vi "Shock&Dyanamics Laboratory - DROPBEAR_June2022_Rev3.vi"() -> ()   [LabVIEW 2019] (continued)
                n889 = property on="SG Pair Ch 18" class="Enum (strict)"("DisabledEnum"=w1070) -> ()  [unwired: 2 in, 2 out]
                n890 = property on="SG Pair Ch 16" class="Enum (strict)"("DisabledEnum"=w1072) -> ()  [unwired: 2 in, 2 out]
                n891 = property on="SG Pair Ch 19" class="Enum (strict)"("DisabledEnum"=w1069) -> ()  [unwired: 2 in, 2 out]
                n892 = property on="SG Pair Ch 26" class="Enum (strict)"("DisabledEnum"=w1061) -> ()  [unwired: 2 in, 2 out]
                n893 = property on="SG Pair Ch 17" class="Enum (strict)"("DisabledEnum"=w1071) -> ()  [unwired: 2 in, 2 out]
                n894 = property on="SG Pair Ch 24" class="Enum (strict)"("DisabledEnum"=w1059) -> ()  [unwired: 2 in, 2 out]
                n895 = property on="SG Pair Ch 27" class="Enum (strict)"("DisabledEnum"=w1062) -> ()  [unwired: 2 in, 2 out]
                n896 = property on="SG Pair Ch 25" class="Enum (strict)"("DisabledEnum"=w1060) -> ()  [unwired: 2 in, 2 out]
                n897 = property on="SG Pair Ch 22" class="Enum (strict)"("DisabledEnum"=w1057) -> ()  [unwired: 2 in, 2 out]
                n898 = property on="SG Pair Ch 30" class="Enum (strict)"("DisabledEnum"=w1065) -> ()  [unwired: 2 in, 2 out]
                n899 = property on="SG Pair Ch 31" class="Enum (strict)"("DisabledEnum"=w1066) -> ()  [unwired: 2 in, 2 out]
                n900 = property on="SG Pair Ch 23" class="Enum (strict)"("DisabledEnum"=w1058) -> ()  [unwired: 2 in, 2 out]
                n901 = property on="SG Pair Ch 28" class="Enum (strict)"("DisabledEnum"=w1063) -> ()  [unwired: 2 in, 2 out]
                n902 = property on="SG Pair Ch 29" class="Enum (strict)"("DisabledEnum"=w1064) -> ()  [unwired: 2 in, 2 out]
                n903 = property on="SG Pair Ch 20" class="Enum (strict)"("DisabledEnum"=w1055) -> ()  [unwired: 2 in, 2 out]
                n904 = property on="SG Pair Ch 21" class="Enum (strict)"("DisabledEnum"=w1056) -> ()  [unwired: 2 in, 2 out]
              }
              event "SG Pair Ch 0", "SG Pair Ch 1", "SG Pair Ch 2", "SG Pair Ch 3", "SG Pair Ch 4", "SG Pair Ch 5", "SG Pair Ch 6", "SG Pair Ch 7", "SG Pair Ch 8", "SG Pair Ch 9", "SG Pair Ch 10", "SG Pair Ch 11", "SG Pair Ch 12", "SG Pair Ch 13", "SG Pair Ch 14", "SG Pair Ch 15", "SG Pair Ch 16", "SG Pair Ch 17", "SG Pair Ch 18", "SG Pair Ch 19", "SG Pair Ch 20", "SG Pair Ch 21", "SG Pair Ch 22", "SG Pair Ch 23", "SG Pair Ch 24", "SG Pair Ch 31", "SG Pair Ch 30", "SG Pair Ch 29", "SG Pair Ch 28", "SG Pair Ch 27", "SG Pair Ch 26", "SG Pair Ch 25": Value Change {
                # "Need to prevent choosing channels to pair if they are not strain, prevent choosing same channel or channel that is already choosen\nprevent pairing channels if they are not turned on - these errors should be before execution!"
                n905 = event-data() -> ()  [unwired: 1 in, 6 out]
                n906 = property on="SG Pair Ch 29" class="Enum (strict)"() -> ("Value"=w1186:T38)  [unwired: 2 in, 2 out]
                n907 = property on="SG Pair Ch 28" class="Enum (strict)"() -> ("Value"=w1187:T37)  [unwired: 2 in, 2 out]
                n908 = property on="SG Pair Ch 31" class="Enum (strict)"() -> ("Value"=w1184:T40)  [unwired: 2 in, 2 out]
                n909 = property on="SG Pair Ch 25" class="Enum (strict)"() -> ("Value"=w1190:T34)  [unwired: 2 in, 2 out]
                n910 = property on="SG Pair Ch 30" class="Enum (strict)"() -> ("Value"=w1185:T39)  [unwired: 2 in, 2 out]
                n911 = property on="SG Pair Ch 24" class="Enum (strict)"() -> ("Value"=w1191:T33)  [unwired: 2 in, 2 out]
                n912 = property on="SG Pair Ch 27" class="Enum (strict)"() -> ("Value"=w1188:T36)  [unwired: 2 in, 2 out]
                n913 = property on="SG Pair Ch 21" class="Enum (strict)"() -> ("Value"=w1194:T30)  [unwired: 2 in, 2 out]
                n914 = property on="SG Pair Ch 26" class="Enum (strict)"() -> ("Value"=w1189:T35)  [unwired: 2 in, 2 out]
                n915 = property on="SG Pair Ch 20" class="Enum (strict)"() -> ("Value"=w1195:T29)  [unwired: 2 in, 2 out]
                n916 = property on="SG Pair Ch 23" class="Enum (strict)"() -> ("Value"=w1192:T32)  [unwired: 2 in, 2 out]
                n917 = property on="SG Pair Ch 13" class="Enum (strict)"() -> ("Value"=w1202:T22)  [unwired: 2 in, 2 out]
                n918 = property on="SG Pair Ch 17" class="Enum (strict)"() -> ("Value"=w1198:T26)  [unwired: 2 in, 2 out]
                n919 = property on="SG Pair Ch 22" class="Enum (strict)"() -> ("Value"=w1193:T31)  [unwired: 2 in, 2 out]
                n920 = property on="SG Pair Ch 12" class="Enum (strict)"() -> ("Value"=w1203:T21)  [unwired: 2 in, 2 out]
                n921 = property on="SG Pair Ch 15" class="Enum (strict)"() -> ("Value"=w1200:T24)  [unwired: 2 in, 2 out]
                n922 = property on="SG Pair Ch 16" class="Enum (strict)"() -> ("Value"=w1199:T25)  [unwired: 2 in, 2 out]
                n923 = property on="SG Pair Ch 19" class="Enum (strict)"() -> ("Value"=w1196:T28)  [unwired: 2 in, 2 out]
                n924 = property on="SG Pair Ch 9" class="Enum (strict)"() -> ("Value"=w1206:T18)  [unwired: 2 in, 2 out]
                n925 = property on="SG Pair Ch 14" class="Enum (strict)"() -> ("Value"=w1201:T23)  [unwired: 2 in, 2 out]
                n926 = property on="SG Pair Ch 18" class="Enum (strict)"() -> ("Value"=w1197:T27)  [unwired: 2 in, 2 out]
                n927 = property on="SG Pair Ch 8" class="Enum (strict)"() -> ("Value"=w1207:T17)  [unwired: 2 in, 2 out]
                n928 = property on="SG Pair Ch 11" class="Enum (strict)"() -> ("Value"=w1204:T20)  [unwired: 2 in, 2 out]
                n929 = property on="SG Pair Ch 5" class="Enum (strict)"() -> ("Value"=w1210:T14)  [unwired: 2 in, 2 out]
                n930 = property on="SG Pair Ch 10" class="Enum (strict)"() -> ("Value"=w1205:T19)  [unwired: 2 in, 2 out]
                n931 = property on="SG Pair Ch 4" class="Enum (strict)"() -> ("Value"=w1211:T13)  [unwired: 2 in, 2 out]
                n932 = property on="SG Pair Ch 7" class="Enum (strict)"() -> ("Value"=w1208:T16)  [unwired: 2 in, 2 out]
                n933 = property on="SG Pair Ch 1" class="Enum (strict)"() -> ("Value"=w1214:T10)  [unwired: 2 in, 2 out]
                n934 = property on="SG Pair Ch 6" class="Enum (strict)"() -> ("Value"=w1209:T15)  [unwired: 2 in, 2 out]
                n935 = property on="SG Pair Ch 0" class="Enum (strict)"() -> ("Value"=w1215:T9)  [unwired: 2 in, 2 out]
                n936 = property on="SG Pair Ch 3" class="Enum (strict)"() -> ("Value"=w1212:T12)  [unwired: 2 in, 2 out]
                n937 = property on="SG Pair Ch 2" class="Enum (strict)"() -> ("Value"=w1213:T11)  [unwired: 2 in, 2 out]
                n938 = Build Array(w1215, w1214, w1213, w1212, w1211, w1210, w1209, w1208, w1207, w1206, w1205, w1204, w1203, w1202, w1201, w1200, w1199, w1198, w1197, w1196, w1195, w1194, w1193, w1192, w1191, w1190, w1189, w1188, w1187, w1186, w1185, w1184) -> (w1217:u16[])
                n939 = for {
                  tunnel: w1217 -> [w1218] mode=indexing
                  i -> [w1219]
                  n940 = Equal?(x=w1219, y=w1218) -> (x = y?=w1221:bool)
                  n941 = Not(x=w1221) -> (.not. x?=w1220:bool)
                  n942 = case shown="True" w1220 {
                    tunnel: w1219 -> [_ w1224]
                    tunnel: w1218 -> [_ w1223]
                    frame False {
                      # "Add error here - cannot pair a Strain Channel with itself"
                      n943 = One Button Dialog(message="The Strain channel cannot be paired with itself. \nPlease select a different channel.") -> ()  [unwired: 1 in, 1 out]
                    }
                    frame True {
                      n944 = case shown="33" w1223 {
                        tunnel: T42."Disabled and Grayed Out" ("Disabled") -> [w1228 w1230 w1233 w1236 w1239 w1242 w1245 w1248 w1251 w1254 w1257 w1260 w1263 w1266 w1269 w1272 w1275 w1278 w1281 w1284 w1287 w1290 w1293 w1296 w1299 w1302 w1305 w1308 w1311 w1314 w1317 w1320 _ _]
                        tunnel: w1224 -> [w1227 w1229 w1232 w1235 w1238 w1241 w1244 w1247 w1250 w1253 w1256 w1259 w1262 w1265 w1268 w1271 w1274 w1277 w1280 w1283 w1286 w1289 w1292 w1295 w1298 w1301 w1304 w1307 w1310 w1313 w1316 w1319 _ _]
                        frame 0, Default {
                          n945 = property on="SG Pair Ch 0" class="Enum (strict)"("Value"=w1227) -> (error out=w1226:errorcluster)  [unwired: 2 in, 1 out]
                          n946 = property on="SG Pair Ch 0" class="Enum (strict)"(error in=w1226, "DisabledEnum"=w1228) -> ()  [unwired: 1 in, 2 out]
                        }
                        frame 1 {
                          n947 = property on="SG Pair Ch 1" class="Enum (strict)"("Value"=w1229) -> (error out=w1231:errorcluster)  [unwired: 2 in, 1 out]
                          n948 = property on="SG Pair Ch 1" class="Enum (strict)"(error in=w1231, "DisabledEnum"=w1230) -> ()  [unwired: 1 in, 2 out]
                        }
                        frame 2 {
                          n949 = property on="SG Pair Ch 2" class="Enum (strict)"("Value"=w1232) -> (error out=w1234:errorcluster)  [unwired: 2 in, 1 out]
                          n950 = property on="SG Pair Ch 2" class="Enum (strict)"(error in=w1234, "DisabledEnum"=w1233) -> ()  [unwired: 1 in, 2 out]
                        }
                        frame 3 {
                          n951 = property on="SG Pair Ch 3" class="Enum (strict)"("Value"=w1235) -> (error out=w1237:errorcluster)  [unwired: 2 in, 1 out]
                          n952 = property on="SG Pair Ch 3" class="Enum (strict)"(error in=w1237, "DisabledEnum"=w1236) -> ()  [unwired: 1 in, 2 out]
                        }
                        frame 4 {
                          n953 = property on="SG Pair Ch 4" class="Enum (strict)"("Value"=w1238) -> (error out=w1240:errorcluster)  [unwired: 2 in, 1 out]
                          n954 = property on="SG Pair Ch 4" class="Enum (strict)"(error in=w1240, "DisabledEnum"=w1239) -> ()  [unwired: 1 in, 2 out]
                        }
                        frame 5 {
                          n955 = property on="SG Pair Ch 5" class="Enum (strict)"("Value"=w1241) -> (error out=w1243:errorcluster)  [unwired: 2 in, 1 out]
                          n956 = property on="SG Pair Ch 5" class="Enum (strict)"(error in=w1243, "DisabledEnum"=w1242) -> ()  [unwired: 1 in, 2 out]
                        }
                        frame 6 {
                          n957 = property on="SG Pair Ch 6" class="Enum (strict)"("Value"=w1244) -> (error out=w1246:errorcluster)  [unwired: 2 in, 1 out]
                          n958 = property on="SG Pair Ch 6" class="Enum (strict)"(error in=w1246, "DisabledEnum"=w1245) -> ()  [unwired: 1 in, 2 out]
                        }
                        frame 7 {
                          n959 = property on="SG Pair Ch 7" class="Enum (strict)"("Value"=w1247) -> (error out=w1249:errorcluster)  [unwired: 2 in, 1 out]
                          n960 = property on="SG Pair Ch 7" class="Enum (strict)"(error in=w1249, "DisabledEnum"=w1248) -> ()  [unwired: 1 in, 2 out]
                        }
                        frame 8 {
                          n961 = property on="SG Pair Ch 8" class="Enum (strict)"("Value"=w1250) -> (error out=w1252:errorcluster)  [unwired: 2 in, 1 out]
                          n962 = property on="SG Pair Ch 8" class="Enum (strict)"(error in=w1252, "DisabledEnum"=w1251) -> ()  [unwired: 1 in, 2 out]
                        }
                        frame 9 {
                          n963 = property on="SG Pair Ch 9" class="Enum (strict)"("Value"=w1253) -> (error out=w1255:errorcluster)  [unwired: 2 in, 1 out]
                          n964 = property on="SG Pair Ch 9" class="Enum (strict)"(error in=w1255, "DisabledEnum"=w1254) -> ()  [unwired: 1 in, 2 out]
                        }
                        frame 10 {
                          n965 = property on="SG Pair Ch 10" class="Enum (strict)"("Value"=w1256) -> (error out=w1258:errorcluster)  [unwired: 2 in, 1 out]
                          n966 = property on="SG Pair Ch 10" class="Enum (strict)"(error in=w1258, "DisabledEnum"=w1257) -> ()  [unwired: 1 in, 2 out]
                        }
                        frame 11 {
                          n967 = property on="SG Pair Ch 11" class="Enum (strict)"("Value"=w1259) -> (error out=w1261:errorcluster)  [unwired: 2 in, 1 out]
                          n968 = property on="SG Pair Ch 11" class="Enum (strict)"(error in=w1261, "DisabledEnum"=w1260) -> ()  [unwired: 1 in, 2 out]
                        }
                        frame 12 {
                          n969 = property on="SG Pair Ch 12" class="Enum (strict)"("Value"=w1262) -> (error out=w1264:errorcluster)  [unwired: 2 in, 1 out]
                          n970 = property on="SG Pair Ch 12" class="Enum (strict)"(error in=w1264, "DisabledEnum"=w1263) -> ()  [unwired: 1 in, 2 out]
                        }
                        frame 13 {
                          n971 = property on="SG Pair Ch 13" class="Enum (strict)"("Value"=w1265) -> (error out=w1267:errorcluster)  [unwired: 2 in, 1 out]
                          n972 = property on="SG Pair Ch 13" class="Enum (strict)"(error in=w1267, "DisabledEnum"=w1266) -> ()  [unwired: 1 in, 2 out]
                        }
                        frame 14 {
                          n973 = property on="SG Pair Ch 14" class="Enum (strict)"("Value"=w1268) -> (error out=w1270:errorcluster)  [unwired: 2 in, 1 out]
                          n974 = property on="SG Pair Ch 14" class="Enum (strict)"(error in=w1270, "DisabledEnum"=w1269) -> ()  [unwired: 1 in, 2 out]
                        }
                        frame 15 {
                          n975 = property on="SG Pair Ch 15" class="Enum (strict)"("Value"=w1271) -> (error out=w1273:errorcluster)  [unwired: 2 in, 1 out]
                          n976 = property on="SG Pair Ch 15" class="Enum (strict)"(error in=w1273, "DisabledEnum"=w1272) -> ()  [unwired: 1 in, 2 out]
                        }
                        frame 16 {
                          n977 = property on="SG Pair Ch 16" class="Enum (strict)"("Value"=w1274) -> (error out=w1276:errorcluster)  [unwired: 2 in, 1 out]
                          n978 = property on="SG Pair Ch 16" class="Enum (strict)"(error in=w1276, "DisabledEnum"=w1275) -> ()  [unwired: 1 in, 2 out]
                        }
                        frame 17 {
                          n979 = property on="SG Pair Ch 17" class="Enum (strict)"("Value"=w1277) -> (error out=w1279:errorcluster)  [unwired: 2 in, 1 out]
                          n980 = property on="SG Pair Ch 17" class="Enum (strict)"(error in=w1279, "DisabledEnum"=w1278) -> ()  [unwired: 1 in, 2 out]
                        }
                        frame 18 {
                          n981 = property on="SG Pair Ch 18" class="Enum (strict)"("Value"=w1280) -> (error out=w1282:errorcluster)  [unwired: 2 in, 1 out]
                          n982 = property on="SG Pair Ch 18" class="Enum (strict)"(error in=w1282, "DisabledEnum"=w1281) -> ()  [unwired: 1 in, 2 out]
                        }
                        frame 19 {
                          n983 = property on="SG Pair Ch 19" class="Enum (strict)"("Value"=w1283) -> (error out=w1285:errorcluster)  [unwired: 2 in, 1 out]
                          n984 = property on="SG Pair Ch 19" class="Enum (strict)"(error in=w1285, "DisabledEnum"=w1284) -> ()  [unwired: 1 in, 2 out]
                        }
                        frame 20 {
                          n985 = property on="SG Pair Ch 20" class="Enum (strict)"("Value"=w1286) -> (error out=w1288:errorcluster)  [unwired: 2 in, 1 out]
                          n986 = property on="SG Pair Ch 20" class="Enum (strict)"(error in=w1288, "DisabledEnum"=w1287) -> ()  [unwired: 1 in, 2 out]
                        }
                        frame 21 {
                          n987 = property on="SG Pair Ch 21" class="Enum (strict)"("Value"=w1289) -> (error out=w1291:errorcluster)  [unwired: 2 in, 1 out]
                          n988 = property on="SG Pair Ch 21" class="Enum (strict)"(error in=w1291, "DisabledEnum"=w1290) -> ()  [unwired: 1 in, 2 out]
                        }
                        frame 22 {
                          n989 = property on="SG Pair Ch 22" class="Enum (strict)"("Value"=w1292) -> (error out=w1294:errorcluster)  [unwired: 2 in, 1 out]
                          n990 = property on="SG Pair Ch 22" class="Enum (strict)"(error in=w1294, "DisabledEnum"=w1293) -> ()  [unwired: 1 in, 2 out]
                        }
                        frame 23 {
                          n991 = property on="SG Pair Ch 23" class="Enum (strict)"("Value"=w1295) -> (error out=w1297:errorcluster)  [unwired: 2 in, 1 out]
                          n992 = property on="SG Pair Ch 23" class="Enum (strict)"(error in=w1297, "DisabledEnum"=w1296) -> ()  [unwired: 1 in, 2 out]
                        }
                        frame 24 {
                          n993 = property on="SG Pair Ch 24" class="Enum (strict)"("Value"=w1298) -> (error out=w1300:errorcluster)  [unwired: 2 in, 1 out]
                          n994 = property on="SG Pair Ch 24" class="Enum (strict)"(error in=w1300, "DisabledEnum"=w1299) -> ()  [unwired: 1 in, 2 out]
                        }
                        frame 25 {
                          n995 = property on="SG Pair Ch 25" class="Enum (strict)"("Value"=w1301) -> (error out=w1303:errorcluster)  [unwired: 2 in, 1 out]
                          n996 = property on="SG Pair Ch 25" class="Enum (strict)"(error in=w1303, "DisabledEnum"=w1302) -> ()  [unwired: 1 in, 2 out]
                        }
                        frame 26 {
                          n997 = property on="SG Pair Ch 26" class="Enum (strict)"("Value"=w1304) -> (error out=w1306:errorcluster)  [unwired: 2 in, 1 out]
                          n998 = property on="SG Pair Ch 26" class="Enum (strict)"(error in=w1306, "DisabledEnum"=w1305) -> ()  [unwired: 1 in, 2 out]
                        }
                        frame 27 {
                          n999 = property on="SG Pair Ch 27" class="Enum (strict)"("Value"=w1307) -> (error out=w1309:errorcluster)  [unwired: 2 in, 1 out]
                          n1000 = property on="SG Pair Ch 27" class="Enum (strict)"(error in=w1309, "DisabledEnum"=w1308) -> ()  [unwired: 1 in, 2 out]
                        }
                        frame 28 {
                          n1001 = property on="SG Pair Ch 28" class="Enum (strict)"("Value"=w1310) -> (error out=w1312:errorcluster)  [unwired: 2 in, 1 out]
                          n1002 = property on="SG Pair Ch 28" class="Enum (strict)"(error in=w1312, "DisabledEnum"=w1311) -> ()  [unwired: 1 in, 2 out]
                        }
                        frame 29 {
                          n1003 = property on="SG Pair Ch 29" class="Enum (strict)"("Value"=w1313) -> (error out=w1315:errorcluster)  [unwired: 2 in, 1 out]
                          n1004 = property on="SG Pair Ch 29" class="Enum (strict)"(error in=w1315, "DisabledEnum"=w1314) -> ()  [unwired: 1 in, 2 out]
                        }
                        frame 30 {
                          n1005 = property on="SG Pair Ch 30" class="Enum (strict)"("Value"=w1316) -> (error out=w1318:errorcluster)  [unwired: 2 in, 1 out]
                          n1006 = property on="SG Pair Ch 30" class="Enum (strict)"(error in=w1318, "DisabledEnum"=w1317) -> ()  [unwired: 1 in, 2 out]
                        }
                        frame 31 {
                          n1007 = property on="SG Pair Ch 31" class="Enum (strict)"("Value"=w1319) -> (error out=w1321:errorcluster)  [unwired: 2 in, 1 out]
                          n1008 = property on="SG Pair Ch 31" class="Enum (strict)"(error in=w1321, "DisabledEnum"=w1320) -> ()  [unwired: 1 in, 2 out]
                        }
                        frame 32 {
                        }
                        frame 33 {
                        }
                      }
                    }
                  }
                }
              }
              event "Signal Type 0", "Signal Type 1", "Signal Type 2", "Signal Type 3", "Signal Type 4", "Signal Type 5", "Signal Type 6", "Signal Type 7", "Signal Type 8", "Signal Type 9", "Signal Type 10", "Signal Type 11", "Signal Type 12", "Signal Type 13", "Signal Type 14", "Signal Type 15", "Signal Type 16", "Signal Type 17", "Signal Type 18", "Signal Type 19", "Signal Type 20", "Signal Type 21", "Signal Type 22", "Signal Type 23", "Signal Type 24", "Signal Type 25", "Signal Type 26", "Signal Type 27", "Signal Type 28", "Signal Type 29", "Signal Type 30", "Signal Type 31": Value Change {
                n1009 = event-data() -> ()  [unwired: 1 in, 5 out]
                n1010 = property on="Signal Type 23" class="Enum (strict)"() -> ("Value"=w1346:T8)  [unwired: 2 in, 2 out]
                n1011 = property on="Signal Type 21" class="Enum (strict)"() -> ("Value"=w1348:T8)  [unwired: 2 in, 2 out]
                n1012 = property on="Signal Type 20" class="Enum (strict)"() -> ("Value"=w1349:T8)  [unwired: 2 in, 2 out]
                n1013 = property on="Signal Type 22" class="Enum (strict)"() -> ("Value"=w1347:T8)  [unwired: 2 in, 2 out]
                n1014 = property on="Signal Type 26" class="Enum (strict)"() -> ("Value"=w1343:T8)  [unwired: 2 in, 2 out]
                n1015 = property on="Signal Type 1" class="Enum (strict)"() -> ("Value"=w1384:T8)  [unwired: 2 in, 2 out]
                n1016 = property on="Signal Type 6" class="Enum (strict)"() -> ("Value"=w1376:T8)  [unwired: 2 in, 2 out]
                n1017 = property on="Signal Type 7" class="Enum (strict)"() -> ("Value"=w1375:T8)  [unwired: 2 in, 2 out]
                n1018 = property on="Signal Type 19" class="Enum (strict)"() -> ("Value"=w1350:T8)  [unwired: 2 in, 2 out]
                n1019 = property on="Signal Type 5" class="Enum (strict)"() -> ("Value"=w1377:T8)  [unwired: 2 in, 2 out]
                n1020 = property on="Signal Type 0" class="Enum (strict)"() -> ("Value"=w1386:T8)  [unwired: 2 in, 2 out]
                n1021 = property on="Signal Type 2" class="Enum (strict)"() -> ("Value"=w1383:T8)  [unwired: 2 in, 2 out]
                n1022 = property on="Signal Type 3" class="Enum (strict)"() -> ("Value"=w1380:T8)  [unwired: 2 in, 2 out]
                n1023 = property on="Signal Type 4" class="Enum (strict)"() -> ("Value"=w1378:T8)  [unwired: 2 in, 2 out]
                n1024 = property on="Signal Type 9" class="Enum (strict)"() -> ("Value"=w1366:T8)  [unwired: 2 in, 2 out]
                n1025 = property on="Signal Type 8" class="Enum (strict)"() -> ("Value"=w1367:T8)  [unwired: 2 in, 2 out]
                n1026 = property on="Signal Type 13" class="Enum (strict)"() -> ("Value"=w1357:T8)  [unwired: 2 in, 2 out]
                n1027 = property on="Signal Type 30" class="Enum (strict)"() -> ("Value"=w1338:T8)  [unwired: 2 in, 2 out]
                n1028 = property on="Signal Type 10" class="Enum (strict)"() -> ("Value"=w1365:T8)  [unwired: 2 in, 2 out]
                n1029 = property on="Signal Type 25" class="Enum (strict)"() -> ("Value"=w1344:T8)  [unwired: 2 in, 2 out]
                n1030 = property on="Signal Type 29" class="Enum (strict)"() -> ("Value"=w1340:T8)  [unwired: 2 in, 2 out]
                n1031 = property on="Signal Type 11" class="Enum (strict)"() -> ("Value"=w1359:T8)  [unwired: 2 in, 2 out]
                n1032 = property on="Signal Type 12" class="Enum (strict)"() -> ("Value"=w1358:T8)  [unwired: 2 in, 2 out]
                n1033 = property on="Signal Type 24" class="Enum (strict)"() -> ("Value"=w1345:T8)  [unwired: 2 in, 2 out]
                n1034 = property on="Signal Type 15" class="Enum (strict)"() -> ("Value"=w1355:T8)  [unwired: 2 in, 2 out]
                n1035 = property on="Signal Type 31" class="Enum (strict)"() -> ("Value"=w1339:T8)  [unwired: 2 in, 2 out]
                n1036 = property on="Signal Type 27" class="Enum (strict)"() -> ("Value"=w1342:T8)  [unwired: 2 in, 2 out]
                n1037 = property on="Signal Type 16" class="Enum (strict)"() -> ("Value"=w1353:T8)  [unwired: 2 in, 2 out]
                n1038 = property on="Signal Type 17" class="Enum (strict)"() -> ("Value"=w1352:T8)  [unwired: 2 in, 2 out]
                n1039 = property on="Signal Type 18" class="Enum (strict)"() -> ("Value"=w1351:T8)  [unwired: 2 in, 2 out]
                n1040 = property on="Signal Type 14" class="Enum (strict)"() -> ("Value"=w1356:T8)  [unwired: 2 in, 2 out]
                n1041 = property on="Signal Type 28" class="Enum (strict)"() -> ("Value"=w1341:T8)  [unwired: 2 in, 2 out]
                n1042 = case shown="\"Voltage\", Default" w1338 {
                  tunnel: [T42."Enabled" ("Disabled") T42."Disabled and Grayed Out" ("Disabled")] -> w1324
                  frame "Strain" {
                    n1043 = property on="SG Pair 30" class="Bool (strict)"() -> ("Value"=w1392:bool)  [unwired: 2 in, 2 out]
                    n1044 = case shown="True" w1392 {
                      tunnel: [T42."Disabled and Grayed Out" ("Disabled") T42."Enabled" ("Disabled")] -> _
                      frame False {
                      }
                      frame True {
                      }
                    }
                  }
                  frame "Voltage", Default {
                  }
                }
                n1045 = case shown="\"Voltage\", Default" w1339 {
                  tunnel: [T42."Enabled" ("Disabled") T42."Disabled and Grayed Out" ("Disabled")] -> w1325
                  frame "Strain" {
                    n1046 = property on="SG Pair 31" class="Bool (strict)"() -> ("Value"=w1387:bool)  [unwired: 2 in, 2 out]
                    n1047 = case shown="True" w1387 {
                      tunnel: [T42."Disabled and Grayed Out" ("Disabled") T42."Enabled" ("Disabled")] -> _
                      frame False {
                      }
                      frame True {
                      }
                    }
                  }
                  frame "Voltage", Default {
                  }
                }
                n1048 = case shown="\"Voltage\", Default" w1340 {
                  tunnel: [T42."Enabled" ("Disabled") T42."Disabled and Grayed Out" ("Disabled")] -> w1323
                  frame "Strain" {
                    n1049 = property on="SG Pair 29" class="Bool (strict)"() -> ("Value"=w1397:bool)  [unwired: 2 in, 2 out]
                    n1050 = case shown="True" w1397 {
                      tunnel: [T42."Disabled and Grayed Out" ("Disabled") T42."Enabled" ("Disabled")] -> _
                      frame False {
                      }
                      frame True {
                      }
                    }
                  }
                  frame "Voltage", Default {
                  }
                }
                n1051 = case shown="\"Strain\"" w1342 {
                  tunnel: [T42."Enabled" ("Disabled") T42."Disabled and Grayed Out" ("Disabled")] -> w1326
                  frame "Strain" {
                    n1052 = property on="SG Pair 27" class="Bool (strict)"() -> ("Value"=w1407:bool)  [unwired: 2 in, 2 out]
                    n1053 = case shown="True" w1407 {
                      tunnel: [T42."Disabled and Grayed Out" ("Disabled") T42."Enabled" ("Disabled")] -> _
                      frame False {
                      }
                      frame True {
                      }
                    }
                  }
                  frame "Voltage", Default {
                  }
                }
                n1054 = case shown="\"Voltage\", Default" w1341 {
                  tunnel: [T42."Enabled" ("Disabled") T42."Disabled and Grayed Out" ("Disabled")] -> w1322
                  frame "Strain" {
                    n1055 = property on="SG Pair 28" class="Bool (strict)"() -> ("Value"=w1402:bool)  [unwired: 2 in, 2 out]
                    n1056 = case shown="True" w1402 {
                      tunnel: [T42."Disabled and Grayed Out" ("Disabled") T42."Enabled" ("Disabled")] -> _
                      frame False {
                      }
                      frame True {
                      }
                    }
                  }
                  frame "Voltage", Default {
                  }
                }
                n1057 = case shown="\"Strain\"" w1343 {
                  tunnel: [T42."Enabled" ("Disabled") T42."Disabled and Grayed Out" ("Disabled")] -> w1327
                  frame "Strain" {
                    n1058 = property on="SG Pair 26" class="Bool (strict)"() -> ("Value"=w1412:bool)  [unwired: 2 in, 2 out]
                    n1059 = case shown="True" w1412 {
                      tunnel: [T42."Disabled and Grayed Out" ("Disabled") T42."Enabled" ("Disabled")] -> _
                      frame False {
                      }
                      frame True {
                      }
                    }
                  }
                  frame "Voltage", Default {
                  }
                }
                n1060 = case shown="\"Voltage\", Default" w1344 {
                  tunnel: [T42."Enabled" ("Disabled") T42."Disabled and Grayed Out" ("Disabled")] -> w1328
                  frame "Strain" {
                    n1061 = property on="SG Pair 25" class="Bool (strict)"() -> ("Value"=w1417:bool)  [unwired: 2 in, 2 out]
                    n1062 = case shown="True" w1417 {
                      tunnel: [T42."Disabled and Grayed Out" ("Disabled") T42."Enabled" ("Disabled")] -> _
                      frame False {
                      }
                      frame True {
                      }
                    }
                  }
                  frame "Voltage", Default {
                  }
                }
                n1063 = case shown="\"Strain\"" w1366 {
                  tunnel: [T42."Enabled" ("Disabled") T42."Disabled and Grayed Out" ("Disabled")] -> w1369
                  frame "Strain" {
                    n1064 = property on="SG Pair 9" class="Bool (strict)"() -> ("Value"=w1497:bool)  [unwired: 2 in, 2 out]
                    n1065 = case shown="True" w1497 {
                      tunnel: [T42."Disabled and Grayed Out" ("Disabled") T42."Enabled" ("Disabled")] -> _
                      frame False {
                      }
                      frame True {
                      }
                    }
                  }
                  frame "Voltage", Default {
                  }
                }
                n1066 = case shown="\"Voltage\", Default" w1345 {
                  tunnel: [T42."Enabled" ("Disabled") T42."Disabled and Grayed Out" ("Disabled")] -> w1329
                  frame "Strain" {
                    n1067 = property on="SG Pair 24" class="Bool (strict)"() -> ("Value"=w1422:bool)  [unwired: 2 in, 2 out]
                    n1068 = case shown="True" w1422 {
                      tunnel: [T42."Disabled and Grayed Out" ("Disabled") T42."Enabled" ("Disabled")] -> _
                      frame False {
                      }
                      frame True {
                      }
                    }
                  }
                  frame "Voltage", Default {
                  }
                }
                n1069 = case shown="\"Strain\"" w1367 {
                  tunnel: [T42."Enabled" ("Disabled") T42."Disabled and Grayed Out" ("Disabled")] -> w1370
                  frame "Strain" {
                    n1070 = property on="SG Pair 8" class="Bool (strict)"() -> ("Value"=w1502:bool)  [unwired: 2 in, 2 out]
                    n1071 = case shown="True" w1502 {
                      tunnel: [T42."Disabled and Grayed Out" ("Disabled") T42."Enabled" ("Disabled")] -> _
                      frame False {
                      }
                      frame True {
                      }
                    }
                  }
                  frame "Voltage", Default {
                  }
                }
                n1072 = case shown="\"Voltage\", Default" w1346 {
                  tunnel: [T42."Enabled" ("Disabled") T42."Disabled and Grayed Out" ("Disabled")] -> w1330
                  frame "Strain" {
                    n1073 = property on="SG Pair 23" class="Bool (strict)"() -> ("Value"=w1427:bool)  [unwired: 2 in, 2 out]
                    n1074 = case shown="True" w1427 {
                      tunnel: [T42."Disabled and Grayed Out" ("Disabled") T42."Enabled" ("Disabled")] -> _
                      frame False {
                      }
                      frame True {
                      }
                    }
                  }
                  frame "Voltage", Default {
                  }
                }
                n1075 = case shown="\"Strain\"" w1378 {
                  tunnel: [T42."Enabled" ("Disabled") T42."Disabled and Grayed Out" ("Disabled")] -> w1371
                  frame "Strain" {
                    n1076 = property on="SG Pair 4" class="Bool (strict)"() -> ("Value"=w1522:bool)  [unwired: 2 in, 2 out]
                    n1077 = case shown="True" w1522 {
                      tunnel: [T42."Disabled and Grayed Out" ("Disabled") T42."Enabled" ("Disabled")] -> _
                      frame False {
                      }
                      frame True {
                      }
                    }
                  }
                  frame "Voltage", Default {
                  }
                }
                n1078 = case shown="\"Strain\"" w1377 {
                  tunnel: [T42."Enabled" ("Disabled") T42."Disabled and Grayed Out" ("Disabled")] -> w1372
                  frame "Strain" {
                    n1079 = property on="SG Pair 5" class="Bool (strict)"() -> ("Value"=w1517:bool)  [unwired: 2 in, 2 out]
                    n1080 = case shown="True" w1517 {
                      tunnel: [T42."Disabled and Grayed Out" ("Disabled") T42."Enabled" ("Disabled")] -> _
                      frame False {
                      }
                      frame True {
                      }
                    }
                  }
                  frame "Voltage", Default {
                  }
                }
                n1081 = case shown="\"Strain\"" w1375 {
                  tunnel: [T42."Enabled" ("Disabled") T42."Disabled and Grayed Out" ("Disabled")] -> w1374
                  frame "Strain" {
                    n1082 = property on="SG Pair 7" class="Bool (strict)"() -> ("Value"=w1507:bool)  [unwired: 2 in, 2 out]
                    n1083 = case shown="True" w1507 {
                      tunnel: [T42."Disabled and Grayed Out" ("Disabled") T42."Enabled" ("Disabled")] -> _
                      frame False {
                      }
                      frame True {
                      }
                    }
                  }
                  frame "Voltage", Default {
                  }
                }
                n1084 = case shown="\"Strain\"" w1358 {
                  tunnel: [T42."Enabled" ("Disabled") T42."Disabled and Grayed Out" ("Disabled")] -> w1363
                  frame "Strain" {
                    n1085 = property on="SG Pair 12" class="Bool (strict)"() -> ("Value"=w1482:bool)  [unwired: 2 in, 2 out]
                    n1086 = case shown="True" w1482 {
                      tunnel: [T42."Disabled and Grayed Out" ("Disabled") T42."Enabled" ("Disabled")] -> _
                      frame False {
                      }
                      frame True {
                      }
                    }
                  }
                  frame "Voltage", Default {
                  }
                }
                n1087 = case shown="\"Voltage\", Default" w1348 {
                  tunnel: [T42."Enabled" ("Disabled") T42."Disabled and Grayed Out" ("Disabled")] -> w1332
                  frame "Strain" {
                    n1088 = property on="SG Pair 21" class="Bool (strict)"() -> ("Value"=w1437:bool)  [unwired: 2 in, 2 out]
                    n1089 = case shown="True" w1437 {
                      tunnel: [T42."Disabled and Grayed Out" ("Disabled") T42."Enabled" ("Disabled")] -> _
                      frame False {
                      }
                      frame True {
                      }
                    }
                  }
                  frame "Voltage", Default {
                  }
                }
                n1090 = case shown="\"Voltage\", Default" w1347 {
                  tunnel: [T42."Enabled" ("Disabled") T42."Disabled and Grayed Out" ("Disabled")] -> w1331
                  frame "Strain" {
                    n1091 = property on="SG Pair 22" class="Bool (strict)"() -> ("Value"=w1432:bool)  [unwired: 2 in, 2 out]
                    n1092 = case shown="True" w1432 {
                      tunnel: [T42."Disabled and Grayed Out" ("Disabled") T42."Enabled" ("Disabled")] -> _
                      frame False {
                      }
                      frame True {
                      }
                    }
                  }
                  frame "Voltage", Default {
                  }
                }
                n1093 = case shown="\"Strain\"" w1365 {
                  tunnel: [T42."Enabled" ("Disabled") T42."Disabled and Grayed Out" ("Disabled")] -> w1368
                  frame "Strain" {
                    n1094 = property on="SG Pair 10" class="Bool (strict)"() -> ("Value"=w1492:bool)  [unwired: 2 in, 2 out]
                    n1095 = case shown="True" w1492 {
                      tunnel: [T42."Disabled and Grayed Out" ("Disabled") T42."Enabled" ("Disabled")] -> _
                      frame False {
                      }
                      frame True {
                      }
                    }
                  }
                  frame "Voltage", Default {
                  }
                }
                n1096 = case shown="\"Strain\"" w1359 {
                  tunnel: [T42."Enabled" ("Disabled") T42."Disabled and Grayed Out" ("Disabled")] -> w1364
                  frame "Strain" {
                    n1097 = property on="SG Pair 11" class="Bool (strict)"() -> ("Value"=w1487:bool)  [unwired: 2 in, 2 out]
                    n1098 = case shown="True" w1487 {
                      tunnel: [T42."Disabled and Grayed Out" ("Disabled") T42."Enabled" ("Disabled")] -> _
                      frame False {
                      }
                      frame True {
                      }
                    }
                  }
                  frame "Voltage", Default {
                  }
                }
                n1099 = case shown="\"Strain\"" w1357 {
                  tunnel: [T42."Enabled" ("Disabled") T42."Disabled and Grayed Out" ("Disabled")] -> w1362
                  frame "Strain" {
                    n1100 = property on="SG Pair 13" class="Bool (strict)"() -> ("Value"=w1477:bool)  [unwired: 2 in, 2 out]
                    n1101 = case shown="True" w1477 {
                      tunnel: [T42."Disabled and Grayed Out" ("Disabled") T42."Enabled" ("Disabled")] -> _
                      frame False {
                      }
                      frame True {
                      }
                    }
                  }
                  frame "Voltage", Default {
                  }
                }
                n1102 = case shown="\"Strain\"" w1351 {
                  tunnel: [T42."Enabled" ("Disabled") T42."Disabled and Grayed Out" ("Disabled")] -> w1335
                  frame "Strain" {
                    n1103 = property on="SG Pair 18" class="Bool (strict)"() -> ("Value"=w1452:bool)  [unwired: 2 in, 2 out]
                    n1104 = case shown="True" w1452 {
                      tunnel: [T42."Disabled and Grayed Out" ("Disabled") T42."Enabled" ("Disabled")] -> _
                      frame False {
                      }
                      frame True {
                      }
                    }
                  }
                  frame "Voltage", Default {
                  }
                }
                n1105 = case shown="\"Strain\"" w1380 {
                  tunnel: [T42."Enabled" ("Disabled") T42."Disabled and Grayed Out" ("Disabled")] -> w1379
                  frame "Strain" {
                    n1106 = property on="SG Pair 3" class="Bool (strict)"() -> ("Value"=w1527:bool)  [unwired: 2 in, 2 out]
                    n1107 = case shown="True" w1527 {
                      tunnel: [T42."Disabled and Grayed Out" ("Disabled") T42."Enabled" ("Disabled")] -> _
                      frame False {
                      }
                      frame True {
                      }
                    }
                  }
                  frame "Voltage", Default {
                  }
                }
                n1108 = case shown="\"Voltage\", Default" w1349 {
                  tunnel: [T42."Enabled" ("Disabled") T42."Disabled and Grayed Out" ("Disabled")] -> w1333
                  frame "Strain" {
                    n1109 = property on="SG Pair 20" class="Bool (strict)"() -> ("Value"=w1442:bool)  [unwired: 2 in, 2 out]
                    n1110 = case shown="True" w1442 {
                      tunnel: [T42."Disabled and Grayed Out" ("Disabled") T42."Enabled" ("Disabled")] -> _
                      frame False {
                      }
                      frame True {
                      }
                    }
                  }
                  frame "Voltage", Default {
                  }
                }
                n1111 = case shown="\"Strain\"" w1356 {
                  tunnel: [T42."Enabled" ("Disabled") T42."Disabled and Grayed Out" ("Disabled")] -> w1361
                  frame "Strain" {
                    n1112 = property on="SG Pair 14" class="Bool (strict)"() -> ("Value"=w1472:bool)  [unwired: 2 in, 2 out]
                    n1113 = case shown="True" w1472 {
